vi "Read Address.vi"(8 "error in (no error)":errorcluster, 11 "CommHandlerBase in":refnum<class "CommHandlerBase.lvclass">) -> (0 "error out":errorcluster, 2 "Address":string, 3 "CommHandlerBase out":refnum<class "CommHandlerBase.lvclass">)   [LabVIEW 2021, in "wamplv.lvlib" / "CommHandlerBase.lvclass"]
uses:
  CommHandlerBase.lvclass
  CommHandlerBase.lvclass/CommHandlerBase.ctl
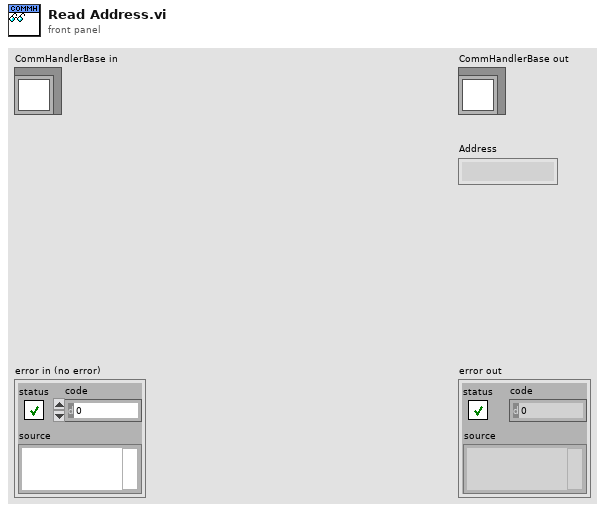
[diagram p1: front panel]
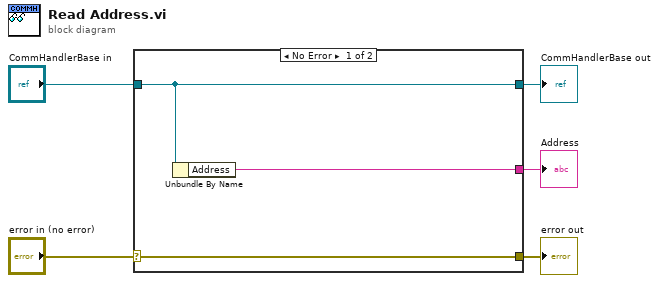
[diagram p0: block diagram]
diagram:
  n1 = case shown="No Error" "error in (no error)" {
    selector: "error in (no error)" -> [w8 w9]
    tunnel: [w8 w9] -> w4
    tunnel: [w7 w10] -> w2
    tunnel: "CommHandlerBase in" -> [w7 w10]
    tunnel: [w6 _] -> w1
    frame No Error {
      n2 = Unbundle By Name(w7) -> ("Address"=w6:string)
    }
    frame Error {
    }
  }
  "error out" <- w4
  "CommHandlerBase out" <- w2
  "Address" <- w1
